vi "Cmd2.vi"(8 "error in (no error)":errorcluster, 11 "VISA Refnum in":refnum<visa-resource-name>) -> (0 "error out":errorcluster, 1 "return count":u32, 3 "VISA Refnum out":refnum<visa-resource-name>)   [LabVIEW 2020]
panel:
  out "time string":string
  out "date string":string
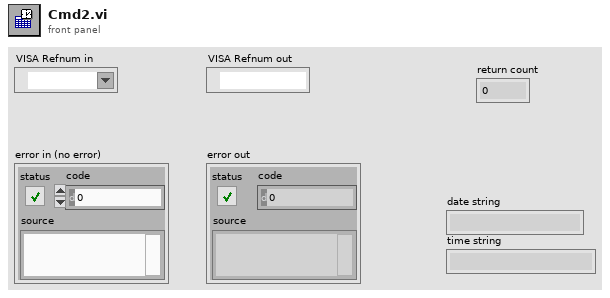
[diagram p1: front panel]
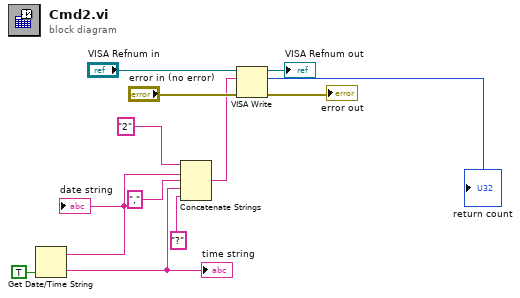
[diagram p0: block diagram]
diagram:
  n1 = Get Date/Time String(want seconds? (F)=TRUE) -> (date string=w9:string, time string=w7:string)  [unwired: 2 in]
  "date string" <- w9
  "time string" <- w7
  n2 = Concatenate Strings("2" ("string"), w9, "," ("string"), w7, "?" ("string")) -> (w5:string)
  n3 = VISA Write(VISA resource name="VISA Refnum in", write buffer=w5, error in (no error)="error in (no error)") -> (VISA resource name out=→"VISA Refnum out":refnum<visa-resource-name>, return count=→"return count":u32, error out=→"error out":errorcluster)
